vi "RANGE Update Accuracy Settings.vi"(0 "Start Up File in":string[][](array[string]), 1 "Meter Accuracy Option 1":T1, 2 "Meter Accuracy Option 2":T1, 3 "Meter Accuracy Option 3":T1, 4 "Meter Accuracy Option 4":T1, 5 "Error In":errorcluster, 7 "Meter Accuracy Option 5":T1, 9 "Meter Accuracy Option 6":T1) -> (14 "Start Up File out":string[][](array[string]), 19 "Error Out":errorcluster)   [LabVIEW 2018]
uses:
  Drivers/Omega FMA-1600A Series Gas Flow Meter/Type Definitions/FMA1600A Meter Accuracy Options.ctl
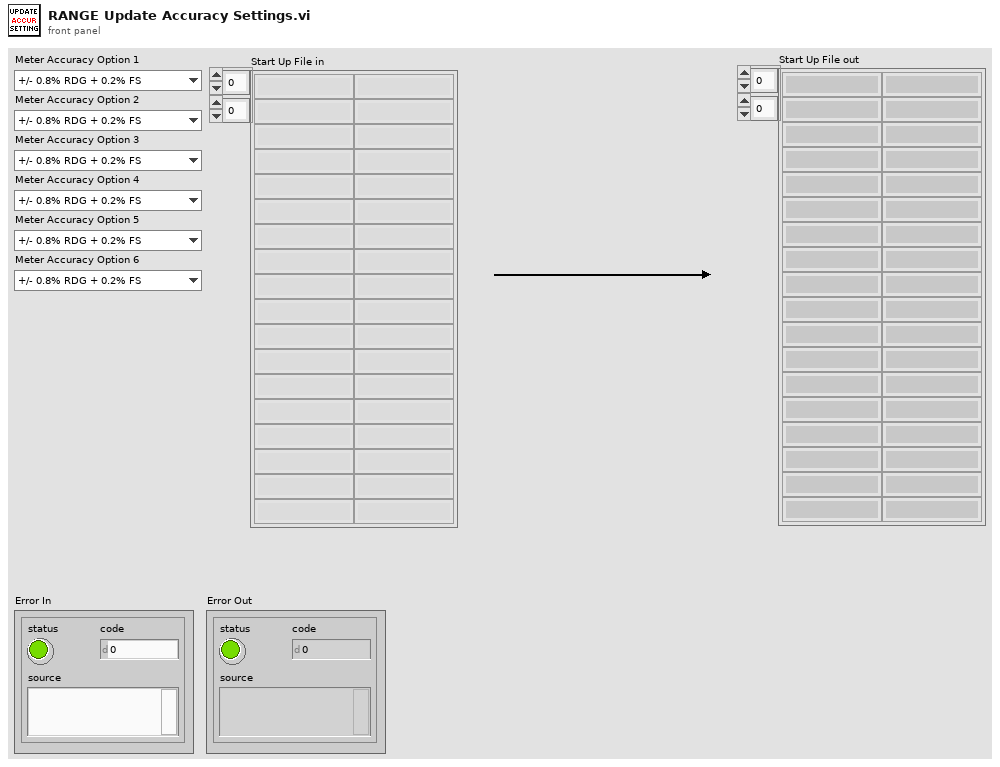
[diagram p1: front panel]
types:
  T1 = typedef "FMA1600A Meter Accuracy Options.ctl" = enum16{"+/- 0.8% RDG + 0.2% FS", "+/- 0.4% RDG + 0.2% FS"}
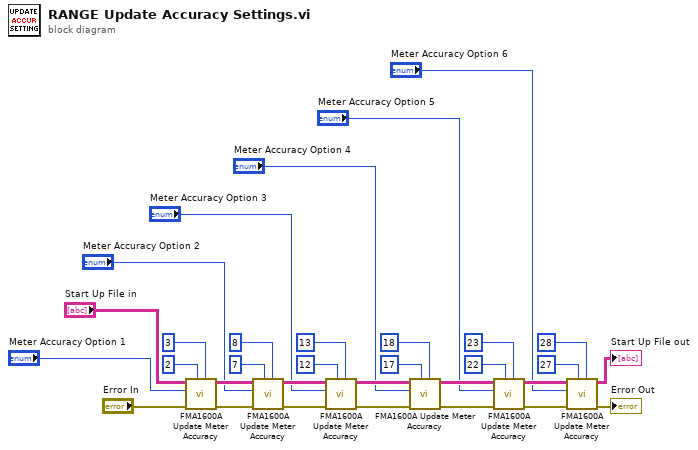
[diagram p0: block diagram]
diagram:
  n1 = call "FMA1600A Update Meter Accuracy.vi"("Full Scale Index"=3, "Reading Index"=2, "Error In"="Error In", "Meter Accuracy Option 1"="Meter Accuracy Option 1", "Start Up File in in"="Start Up File in") -> ("Error Out"=w11:errorcluster, "Start Up File out"=w28:string[][])  [unwired: 5 in]
  n2 = call "FMA1600A Update Meter Accuracy.vi"("Full Scale Index"=8, "Reading Index"=7, "Error In"=w11, "Meter Accuracy Option 1"="Meter Accuracy Option 2", "Start Up File in in"=w28) -> ("Error Out"=w10:errorcluster, "Start Up File out"=w25:string[][])  [unwired: 5 in]
  n3 = call "FMA1600A Update Meter Accuracy.vi"("Full Scale Index"=13, "Reading Index"=12, "Error In"=w10, "Meter Accuracy Option 1"="Meter Accuracy Option 3", "Start Up File in in"=w25) -> ("Error Out"=w9:errorcluster, "Start Up File out"=w20:string[][])  [unwired: 5 in]
  n4 = call "FMA1600A Update Meter Accuracy.vi"("Full Scale Index"=18, "Reading Index"=17, "Error In"=w9, "Meter Accuracy Option 1"="Meter Accuracy Option 4", "Start Up File in in"=w20) -> ("Error Out"=w19:errorcluster, "Start Up File out"=w18:string[][])  [unwired: 5 in]
  n5 = call "FMA1600A Update Meter Accuracy.vi"("Full Scale Index"=23, "Reading Index"=22, "Error In"=w19, "Meter Accuracy Option 1"="Meter Accuracy Option 5", "Start Up File in in"=w18) -> ("Error Out"=w14:errorcluster, "Start Up File out"=w15:string[][])  [unwired: 5 in]
  n6 = call "FMA1600A Update Meter Accuracy.vi"("Full Scale Index"=28, "Reading Index"=27, "Error In"=w14, "Meter Accuracy Option 1"="Meter Accuracy Option 6", "Start Up File in in"=w15) -> ("Error Out"=→"Error Out":errorcluster, "Start Up File out"=→"Start Up File out":string[][])  [unwired: 5 in]
